vi "OpenGitRemote.vi"() -> ()   [LabVIEW 2020]
uses:
  <userlib>/_OpenG.lib/file/file.llb/Valid Path - Traditional__ogtk.vi
  <userlib>/_OpenG.lib/file/file.llb/openg_file.lvlib
panel:
  out "GitRootDetected?":bool
  out "GitRootPath":path
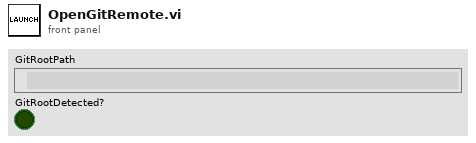
[diagram p1: front panel]
types:
  T1 = enum32{"Invalid", "Standard", "Closed", "Hidden", "Minimized", "Maximized"}
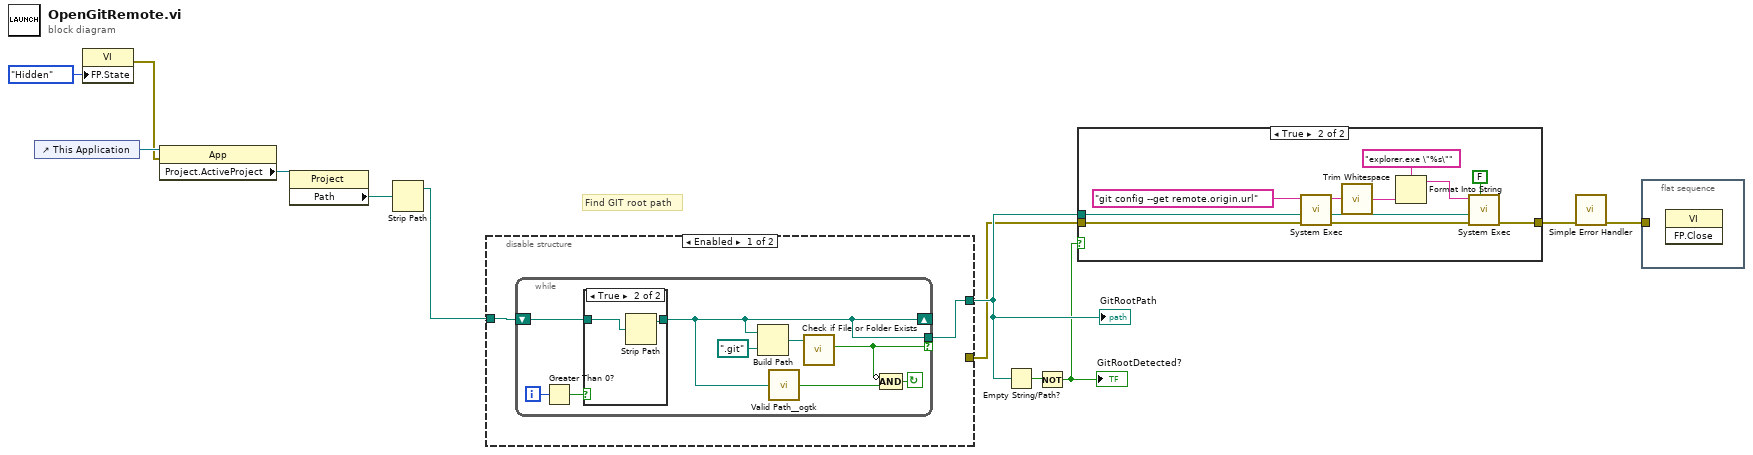
[diagram p0: block diagram]
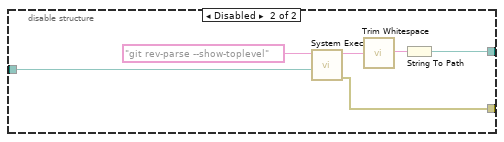
[diagram p4: hidden frame]
diagram:
  # "Find GIT root path"
  n1 = control-ref of="This Application"() -> (w11:refnum<vi>)
  n2 = property class="VI"("FP.State"=T1."Hidden" ("Front Panel Window:State")) -> (error out=w6:errorcluster)  [unwired: 2 in, 1 out]
  n3 = property class="App"(reference=w11, error in=w6) -> ("Project.ActiveProject"=w10:refnum<vi>)  [unwired: 2 out]
  n4 = property class="Project"(reference=w10) -> ("Path"=w9:path)  [unwired: 1 in, 2 out]
  n5 = Strip Path(path=w9) -> (stripped path=w4:path)  [unwired: 1 out]
  n6 = disable-structure shown="Enabled" {
    disable-tunnel: w4 -> [w14 w27]
    disable-tunnel: [w13 w28] -> w3
    disable-tunnel: [_ w29] -> w2
    frame Enabled {
      n7 = while {
        shift-right: [w18] -> _
        shift-left: w14 -> [w19]
        tunnel: [w18] -> w13 if=w15
        i -> [w21]
        stop <- w17 continue-if-true
        n8 = Greater Than 0?(x=w21) -> (x > 0?=w20:bool)
        n9 = case shown="True" w20 {
          tunnel: [w24 w25] -> w18
          tunnel: w19 -> [w24 w26]
          frame False {
          }
          frame True {
            n10 = Strip Path(path=w26) -> (stripped path=w25:path)  [unwired: 1 out]
          }
        }
        n11 = Build Path(base path=w18, name or relative path=path ".git") -> (appended path=w23:path)
        n12 = call-poly <userlib>:"Valid Path__ogtk.vi"("path"=w18) -> ("valid"=w16:bool)
        n13 = call <vilib>:"Check if File or Folder Exists.vi"("path"=w23) -> ("file or folder exists?"=w15:bool)  [unwired: 8 in, 2 out]
        n14 = Compound Arithmetic op=AND(invert w15, w16) -> (w17:bool)
      }
    }
    frame Disabled {
      n15 = call <vilib>:"System Exec.vi"("working directory"=w27, "command line"="git rev-parse --show-toplevel" ("key")) -> ("error out"=w29:errorcluster, "standard output"=w31:string)  [unwired: 6 in, 2 out]
      n16 = call <vilib>:"Trim Whitespace.vi"("string"=w31) -> ("trimmed string"=w32:string)  [unwired: 1 in]
      n17 = String To Path(string=w32) -> (path=w28:path)
    }
  }
  "GitRootPath" <- w3
  n18 = Empty String/Path?(string/path=w3) -> (empty?=w5:bool)
  n19 = Not(x=w5) -> (.not. x?=w1:bool)
  "GitRootDetected?" <- w1
  n20 = case shown="True" w1 {
    tunnel: [w33 w43] -> w12
    tunnel: w3 -> [_ w38]
    tunnel: w2 -> [w33 w37]
    frame False {
    }
    frame True {
      n21 = call <vilib>:"System Exec.vi"("error in (no error)"=w37, "working directory"=w38, "command line"="git config --get remote.origin.url" ("key")) -> ("error out"=w36:errorcluster, "standard output"=w35:string)  [unwired: 5 in, 2 out]
      n22 = call <vilib>:"Trim Whitespace.vi"("string"=w35) -> ("trimmed string"=w34:string)  [unwired: 1 in]
      n23 = Format Into String(format string="explorer.exe \"%s\"", w34) -> (resulting string=w41:string)  [unwired: 2 in, 1 out]
      n24 = call <vilib>:"System Exec.vi"("wait until completion? (T)"=FALSE, "error in (no error)"=w36, "working directory"=w38, "command line"=w41) -> ("error out"=w43:errorcluster)  [unwired: 4 in, 3 out]
    }
  }
  n25 = call <vilib>:"Simple Error Handler.vi"("error in (no error)"=w12) -> ("error out"=w8:errorcluster)  [unwired: 4 in, 4 out]
  n26 = flat-sequence {
    tunnel: w8 -> [_]
    frame #0 {
      n27 = invoke class="VI" method="FP.Close"() -> ()  [unwired: 3 in, 3 out]
    }
  }
